vi "dscInit.vi"(8 "error in":errorcluster, 11 "versionIn":u16) -> (0 "error out":errorcluster, 3 "versionOut":u16)   [LabVIEW 2011, in "Diamond Universal Driver.lvlib"]
doc: "Initialize the universal driver. This function must be included at the beginning of any operation which will utilize the unversal driver."
uses:
  Diamond Universal Driver.lvlib
  Controls/error codes.ctl
  Instruments/WL OPC/Support/dlls/dscud.dll
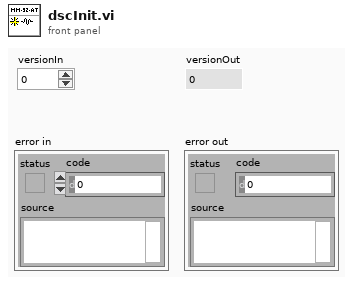
[diagram p1: front panel]
types:
  T1 = typedef "Diamond Universal Driver.lvlib/error codes.ctl" = enum8{"DE_NONE", "DE_HW_FAILURE", "DE_SW_FAILURE", "DE_HW_NOT_SUPPORTED", "DE_SW_NOT_SUPPORTED", "DE_INVALID_PARM", "DE_ALTERNATE_IN_PROGRESS", "DE_NONE_IN_PROGRESS", "DE_BUFFER_ROLLOVER", "DE_INVALID_ERROR_CODE", "DE_ALREADY_PAUSED", "DE_OVERFLOW", "DE_INVALID_FUNC", "DE_DSCUDH_INVALID", "DE_INVALID_BOARD", "DE_BOARD_LIMIT_REACHED", "DE_BOARD_BUSY", "DE_INVALID_WINDRVR_HANDLE", "DE_INVALID_WINDRVR_VERSION", "DE_BAD_WINDRVR_BOARD_INIT", "DE_OPERATION_TIMED_OUT", "DE_INVALID_WINDRVR_KP", "DE_THREAD_FAILURE"}
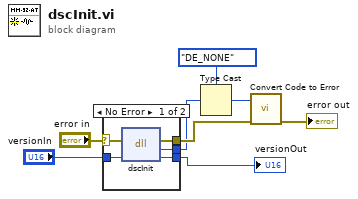
[diagram p0: block diagram]
diagram:
  n1 = case shown="No Error" "error in" {
    selector: "error in" -> [w9 w14]
    tunnel: "versionIn" -> [w13 w15]
    tunnel: [w12 w15] -> w8
    tunnel: [w11 _] -> w3
    tunnel: [w10 w14] -> w5
    frame No Error {
      n2 = dll-call lib="C:/Users/mrichardson/Documents/Web Based Version Control SW/Instruments/WL OPC/Support/dlls/dscud.dll" fn="dscInit"(error in=w9, "version"=w13) -> (error out=w10:errorcluster, "result"=w11:u8, "version"=w12:u16)  [unwired: 2 in, 1 out]
    }
    frame Error {
    }
  }
  "versionOut" <- w8
  n3 = Type Cast(type=error_codes."DE_NONE" ("error codes"), x=w3) -> (*(type *) &x=w2:T1)
  n4 = call "Convert Code to Error.vi"("error in"=w5, "error codes"=w2) -> ("error out"=→"error out":errorcluster)  [unwired: 9 in]
